vi "Measurement Logic.vi"() -> ()   [LabVIEW 2023, in "LabVIEW Bodeplot Summit.lvlib"]
doc: "ML Measurement Logic"
uses:
  LabVIEW Bodeplot Summit.lvlib
  Measurement Configuration.ctl
  <vilib>/MeasurementLink/MeasurementLink Measurement Server/Classes/MeasurementContext/MeasurementContext.lvclass
  Logic/Bode Plot - PXI.lvlib
  Measurement Results.ctl
panel:
  out "Measurement Context out":refnum<class "MeasurementContext.lvclass">
  in  "Measurement Context":refnum<class "MeasurementContext.lvclass">
  out "Measurement Results":T1
  in  "Measurement Configuration":T2={"Start Freq."=1000.0, "Freq. Step"=10.0, "Stop Frequ."=1000000.0, "Amplitude"=1.0, "Timing (ms)"=0, "Vin_signal"="", "Vin_measure"="", "Vout_measure"=""} {"Stop Frequ." format="%#_6p"; "Freq. Step" format="%#_6p"; "Start Freq." format="%#_6p"}
  out "error out":errorcluster
  in  "error in":errorcluster
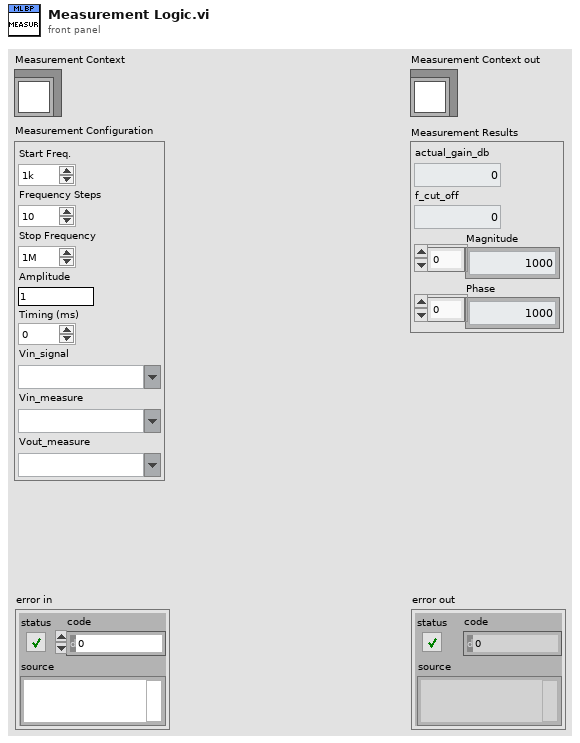
[diagram p1: front panel]
types:
  T1 = typedef "LabVIEW Bodeplot Summit.lvlib/Measurement Results.ctl" = cluster{"actual_gain_db":dbl, "f_cut_off":dbl, "Magnitude":dbl[], "Phase":dbl[]}
  T2 = typedef "LabVIEW Bodeplot Summit.lvlib/Measurement Configuration.ctl" = cluster{"Start Freq.":dbl, "Freq. Step":dbl, "Stop Frequ.":dbl, "Amplitude":dbl, "Timing (ms)":u32, "Vin_signal":string, "Vin_measure":string, "Vout_measure":string}
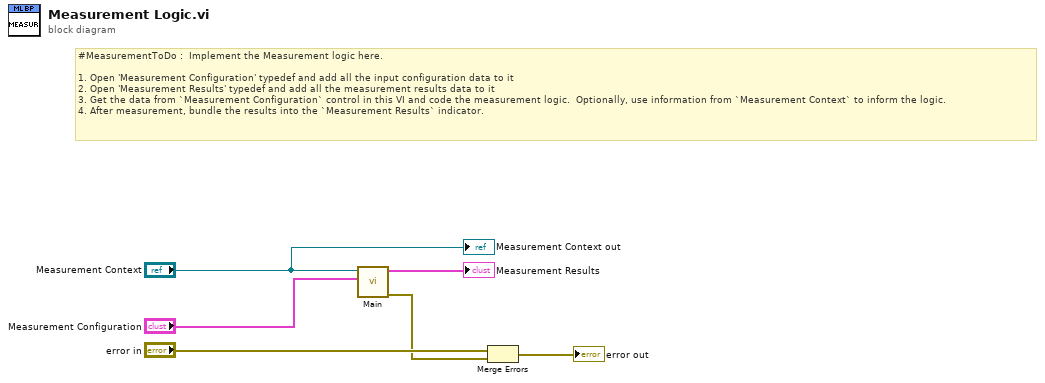
[diagram p0: block diagram]
diagram:
  # "#MeasurementToDo :  Implement the Measurement logic here.\n\n1. Open 'Measurement Configuration' typedef and add all the input configuration data to it\n2. Open 'Measurement Results' typedef and add all the measurement results data to it\n3. Get the data from `Measurement Configuration` control in this VI and code the measurement logic.  Optionally, use information from `Measurement Context` to inform the logic.\n4. After measurement, bundle the results into the `Measurement Results` indicator."
  n1 = call "Main.vi"("Measurement Configuration"="Measurement Configuration", "Measurement Context"="Measurement Context") -> ("error out"=w1:errorcluster, "Results"=→"Measurement Results":T1)  [unwired: 8 in]
  n2 = Merge Errors("error in", w1) -> (→"error out":errorcluster)
  "Measurement Context out" <- "Measurement Context"
